vi "PI_WAV_column_sas.vi"(5 "Attach to wav":bool, 6 "Steps per Scan-line":u16, 7 "Axis Identifier":string, 8 "Amplitude / [mu]":dbl, 9 "Startpos / [mu]":dbl, 10 "Pixel per scan":u16, 11 "Commandset in":string[](array[string])) -> (3 "Commandset out":string[](array[string]))   [LabVIEW 2009]
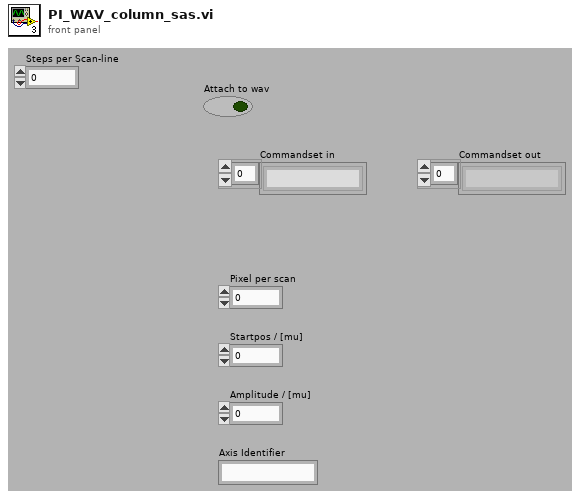
[diagram p1: front panel]
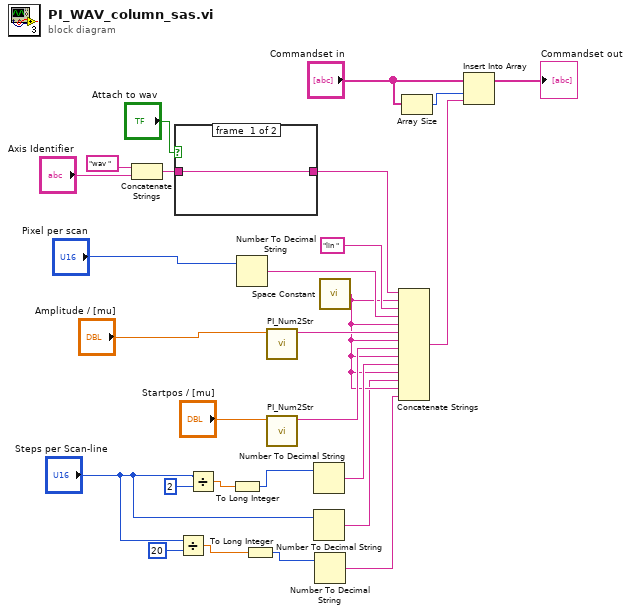
[diagram p0: block diagram]
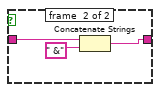
[diagram p2: hidden frame]
diagram:
  n1 = Concatenate Strings("wav " ("new element/subarray"), "Axis Identifier") -> (w14:string)
  n2 = case shown="False" "Attach to wav" {
    tunnel: w14 -> [w28 w31]
    tunnel: [w28 w29] -> w13
    frame #0 {
    }
    frame #1 {
      n3 = Concatenate Strings(w31, " &" ("string")) -> (w29:string)
    }
  }
  n4 = Divide(x="Steps per Scan-line", y=u16 20) -> (x/y=w4:dbl)
  n5 = Divide(x="Steps per Scan-line", y=u16 2) -> (x/y=w8:dbl)
  n6 = To Long Integer(number=w8) -> (32bit integer=w7:i32)
  n7 = Number To Decimal String(number="Pixel per scan") -> (decimal integer string=w21:string)  [unwired: 1 out]
  n8 = To Long Integer(number=w4) -> (32bit integer=w3:i32)
  n9 = call "PI_Num2Str.vi"("x-Position"="Amplitude / [mu]") -> ("String"=w24:string)  [unwired: 10 out]
  n10 = call "PI_Num2Str.vi"("x-Position"="Startpos / [mu]") -> ("String"=w25:string)  [unwired: 10 out]
  n11 = Number To Decimal String(number=w7) -> (decimal integer string=w27:string)  [unwired: 1 out]
  n12 = Number To Decimal String(number="Steps per Scan-line") -> (decimal integer string=w10:string)  [unwired: 1 out]
  n13 = Number To Decimal String(number=w3) -> (decimal integer string=w2:string)  [unwired: 1 out]
  n14 = call <vilib>:"Space Constant.vi"() -> ("String"=w11:string)
  n15 = Concatenate Strings(w13, w11, "lin " ("string"), w21, w11, w24, w11, w25, w11, w27, w11, w10, w11, w2) -> (w22:string)
  n16 = Array Size(array="Commandset in") -> (size(s)=w17:i32)
  n17 = Insert Into Array(array="Commandset in", index=w17, new element=w22) -> (→"Commandset out":string[])
